vi "Write VISAHandle.vi"(8 "error in (no error)":errorcluster, 10 "VISAHandle":refnum<visa-resource-name>, 11 "Keysight335XX in":refnum<class "Keysight335XX.lvclass">) -> (0 "error out":errorcluster, 3 "Keysight335XX out":refnum<class "Keysight335XX.lvclass">)   [LabVIEW 2014, in "FGenPlugins.lvlib" / "Keysight335XX.lvclass"]
uses:
  Keysight335XX.lvclass
  Keysight335XX.lvclass/Keysight335XX.ctl
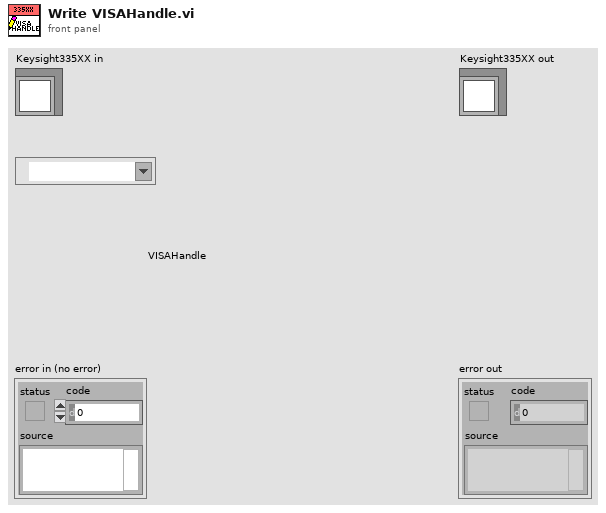
[diagram p1: front panel]
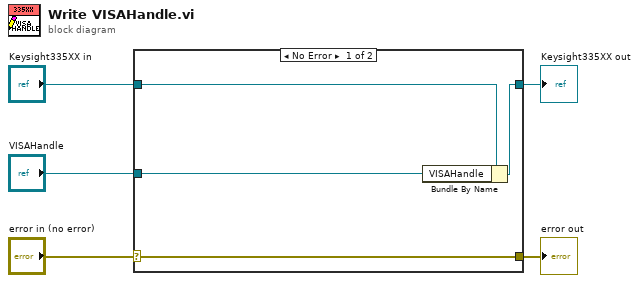
[diagram p0: block diagram]
diagram:
  n1 = case shown="No Error" "error in (no error)" {
    selector: "error in (no error)" -> [w9 w10]
    tunnel: [w9 w10] -> w4
    tunnel: [w7 w11] -> w2
    tunnel: "Keysight335XX in" -> [w8 w11]
    tunnel: "VISAHandle" -> [w6 _]
    frame No Error {
      n2 = Bundle By Name(cluster=w8, "VISAHandle"=w6) -> (w7:refnum<class "Keysight335XX.lvclass">)
    }
    frame Error {
    }
  }
  "error out" <- w4
  "Keysight335XX out" <- w2
